vi "Obtain Request Events.vi"(8 "error in":errorcluster, 10 "Create New? (F)":bool) -> (0 "error out":errorcluster, 2 "PLC Request Events":T1)   [LabVIEW 2024, in "PLC.lvlib"]
doc: "This VI Obtains/Creates the Requests events that will be used for other modules to communicate with the module that owns this VI. These Requests events will be accessed only via Public API methods for this module.\n\n<b>NOTE</b>: The contents of this VI are automatically generated and modified by the <b>Tools > DQMH Consortium > DQMH</b> utilities. Consider using those utilities instead of making your own modifications to this VI.\n_____\nBased on DQMH Dev Tools: Project Template 7.1.0.1503."
uses:
  PLC.lvlib
  Request Events--cluster.ctl
  Stop Argument--cluster.ctl
  Show Panel Argument--cluster.ctl
  Hide Panel Argument--cluster.ctl
  Get Module Execution Status Argument--cluster.ctl
  Show Diagram Argument--cluster.ctl
  set coil value Argument--cluster.ctl
  set register value Argument--cluster.ctl
  read coils Argument--cluster.ctl
  connect Argument--cluster.ctl
panel:
  # "NOTE: The contents of this VI are automatically generated and modified by the Tools > DQMH Consortium > DQMH utilities. Consider using those utilities instead of making your own modifications to this VI."
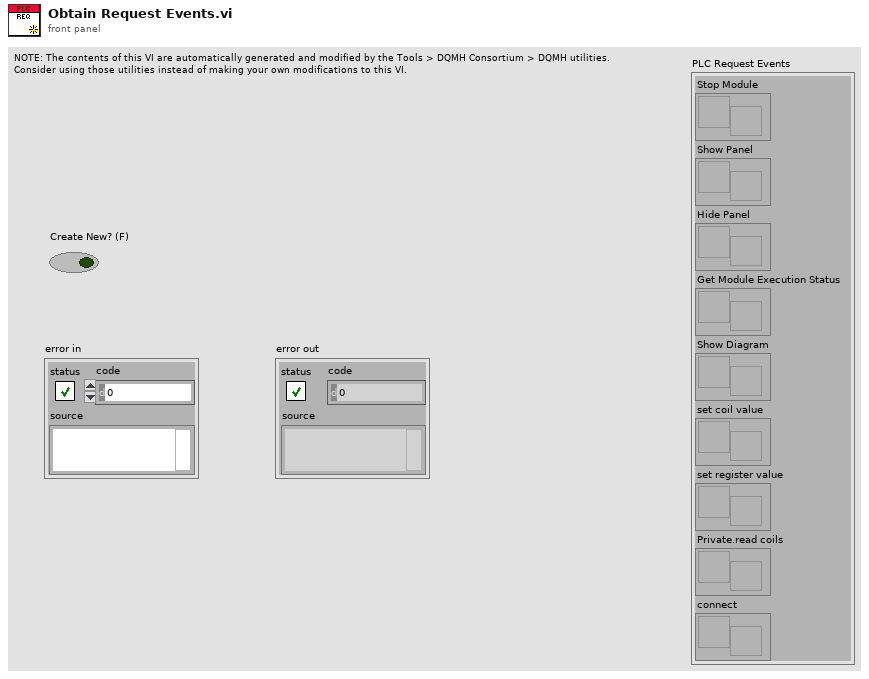
[diagram p1: front panel]
types:
  T1 = typedef "PLC.lvlib/Request Events--cluster.ctl" = cluster{"Stop Module":refnum<user-event>, "Show Panel":refnum<user-event>, "Hide Panel":refnum<user-event>, "Get Module Execution Status":refnum<user-event>, "Show Diagram":refnum<user-event>, "set coil value":refnum<user-event>, "set register value":refnum<user-event>, "Private.read coils":refnum<user-event>, "connect":refnum<user-event>}
  T2 = typedef "PLC.lvlib/connect Argument--cluster.ctl" = cluster{"IP address":string, "Port":dbl}
  T3 = typedef "PLC.lvlib/read coils Argument--cluster.ctl" = cluster{"number of coils to read":dbl}
  T4 = typedef "PLC.lvlib/set register value Argument--cluster.ctl" = cluster{"Register number":u16, "value":dbl}
  T5 = typedef "PLC.lvlib/set coil value Argument--cluster.ctl" = cluster{"ON/OFF":bool, "Ring":u16}
  T6 = typedef "PLC.lvlib/Hide Panel Argument--cluster.ctl" = cluster{"Hide Panel?":bool}
  T7 = typedef "PLC.lvlib/Show Panel Argument--cluster.ctl" = cluster{"Show Panel?":bool}
  T8 = typedef "PLC.lvlib/Show Diagram Argument--cluster.ctl" = cluster{"Debug?":bool}
  T9 = typedef "PLC.lvlib/Get Module Execution Status Argument--cluster.ctl" = cluster{"Running?":bool}
  T10 = typedef "PLC.lvlib/Stop Argument--cluster.ctl" = cluster{"Origin":string, "Exit via Stop Module Req?":bool, "Wait for Module to stop?":bool}
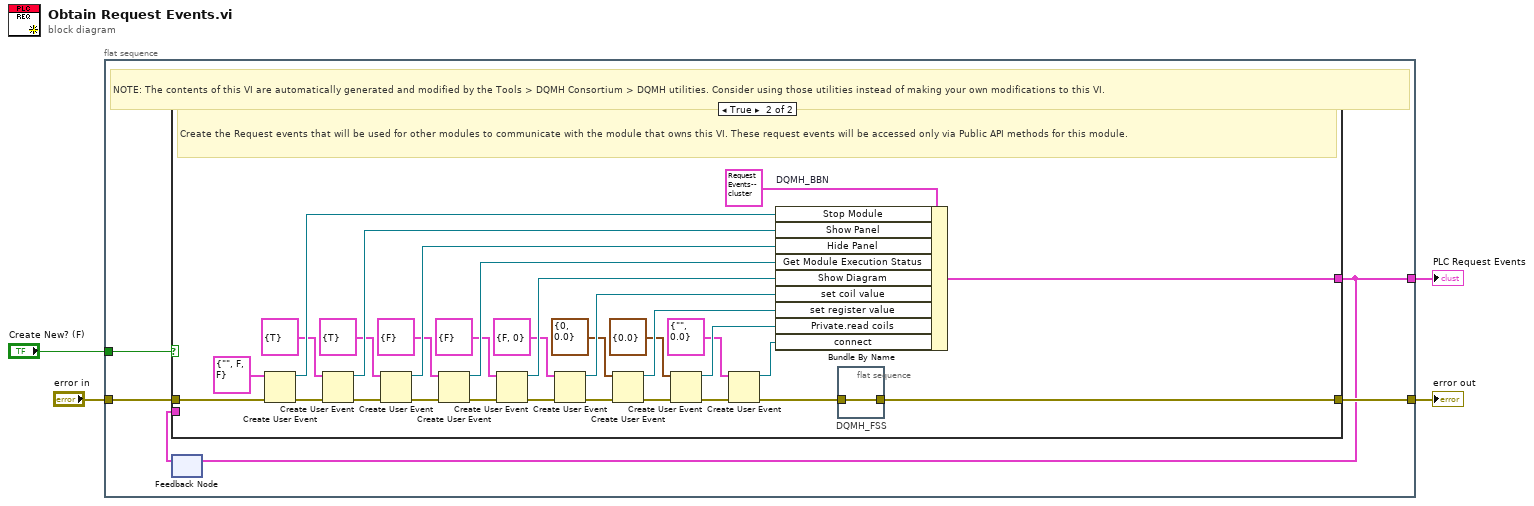
[diagram p0: block diagram]
diagram:
  n1 = flat-sequence {
    tunnel: [w9] -> w4
    tunnel: "error in" -> [w8]
    tunnel: [w6] -> w2
    tunnel: "Create New? (F)" -> [w5]
    frame #0 {
      # "NOTE: The contents of this VI are automatically generated and modified by the Tools > DQMH Consortium > DQMH utilities. Consider using those utilities instead of making your own modifications to this VI."
      n2 = feedback #1() -> (w7:T1)  [unwired: 1 in]
      n3 = case shown="True" w5 {
        tunnel: [w10 w32] -> w9
        tunnel: w8 -> [w10 w42]
        tunnel: [w11 w39] -> w6
        tunnel: w7 -> [w11 _]
        frame False {
          # "Obtain the Request events that were created in a previous call to this VI."
        }
        frame True {
          # "Create the Request events that will be used for other modules to communicate with the module that owns this VI. These request events will be accessed only via Public API methods for this module."
          n4 = Create User Event(user event datatype=T10 {"Origin"="", "Exit via Stop Module Req?"=FALSE, "Wait for Module to stop?"=FALSE} ("Stop Argument"), error in=w42) -> (user event=w40:refnum<user-event>, error out=w37:errorcluster)
          n5 = Create User Event(user event datatype=T7 {"Show Panel?"=TRUE} ("Show Panel Argument"), error in=w37) -> (user event=w36:refnum<user-event>, error out=w35:errorcluster)
          n6 = Create User Event(user event datatype=T6 {"Hide Panel?"=TRUE} ("Hide Panel Argument"), error in=w35) -> (user event=w34:refnum<user-event>, error out=w33:errorcluster)
          n7 = Create User Event(user event datatype=T9 {"Running?"=FALSE} ("Get Module Execution Status Argument"), error in=w33) -> (user event=w30:refnum<user-event>, error out=w31:errorcluster)
          n8 = Create User Event(user event datatype=T8 {"Debug?"=FALSE} ("Show Diagram Argument"), error in=w31) -> (user event=w27:refnum<user-event>, error out=w28:errorcluster)
          n9 = Create User Event(user event datatype=T5 {"ON/OFF"=FALSE, "Ring"=0} ("set coil value Argument"), error in=w28) -> (user event=w22:refnum<user-event>, error out=w23:errorcluster)
          n10 = Create User Event(user event datatype=T4 {"Register number"=0, "value"=0.0} ("set register value Argument"), error in=w23) -> (user event=w19:refnum<user-event>, error out=w20:errorcluster)
          n11 = Create User Event(user event datatype=T3 {"number of coils to read"=0.0} ("read coils Argument"), error in=w20) -> (user event=w16:refnum<user-event>, error out=w17:errorcluster)
          n12 = Create User Event(user event datatype=T2 {"IP address"="", "Port"=0.0} ("connect Argument"), error in=w17) -> (user event=w13:refnum<user-event>, error out=w14:errorcluster)
          n13 = Bundle By Name "DQMH_BBN"(cluster=T1 {"Stop Module"=refnum, "Show Panel"=refnum, "Hide Panel"=refnum, "Get Module Execution Status"=refnum, "Show Diagram"=refnum, "set coil value"=refnum, "set register value"=refnum, "Private.read coils"=refnum, "connect"=refnum} ("output cluster"), "Stop Module"=w40, "Show Panel"=w36, "Hide Panel"=w34, "Get Module Execution Status"=w30, "Show Diagram"=w27, "set coil value"=w22, "set register value"=w19, "Private.read coils"=w16, "connect"=w13) -> (w39:T1)
          n14 = flat-sequence "DQMH_FSS" {
            tunnel: w14 -> [w43]
            tunnel: [w43] -> w32
            frame #0 {
            }
          }
        }
      }
      n15 = feedback-in #1(w6) -> ()
    }
  }
  "PLC Request Events" <- w2
  "error out" <- w4
